vi "launchConnectionListener.vi"(8 "error in (no error)":errorcluster, 11 "BuildServer in":refnum<class "BuildServer.lvclass">) -> (0 "error out":errorcluster, 3 "BuildServer out":refnum<class "BuildServer.lvclass">)   [LabVIEW 2017, in "BuildServer.lvlib" / "BuildServer.lvclass"]
uses:
  BuildServer.lvclass
  C:/Program Files (x86)/National Instruments/LabVIEW 2017/vi.lib/ActorFramework/Actor/Actor.lvclass
  BuildServer.lvclass/BuildServer.ctl
  Communication/Connection Listener/Connection Listener/Connection Listener.lvclass/Connection Listener.ctl
  Communication/Connection Listener/Connection Listener/Read Msg Update.vi
  Communication/Connection Listener/Connection Listener/Connection Listener.lvclass
  <vilib>/ActorFramework/Actor/Actor.lvclass
  Classes/Comm Interface/Comm Interface.lvclass
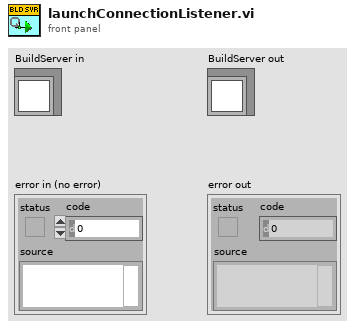
[diagram p1: front panel]
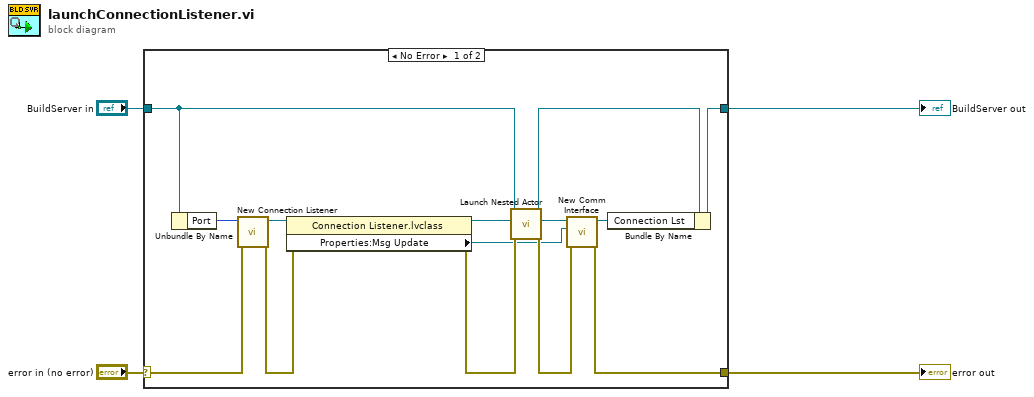
[diagram p0: block diagram]
diagram:
  n1 = case shown="No Error" "error in (no error)" {
    selector: "error in (no error)" -> [w18 w20]
    tunnel: [w10 w20] -> w3
    tunnel: [w14 w19] -> w1
    tunnel: "BuildServer in" -> [w16 w19]
    frame No Error {
      n2 = Unbundle By Name(w16) -> ("Port"=w5:u16)
      n3 = call "New Connection Listener.vi"("error in (no error)"=w18, "Port"=w5) -> ("error out"=w8:errorcluster, "Connection Listener out"=w17:refnum<class "Connection Listener.lvclass">)  [unwired: 8 in]
      n4 = property class="Connection Listener.lvclass"(reference=w17, error in=w8) -> (reference out=w9:refnum<class "Connection Listener.lvclass">, error out=w7:errorcluster, "Properties:Msg Update"=w6:refnum<user-event>)
      n5 = call <vilib>:"Launch Nested Actor.vi"("error in (no error)"=w7, "Nested Actor"=w9, "Caller Actor in"=w16) -> ("error out"=w11:errorcluster, "Nested Actor's Enqueuer"=w13:refnum<class "Message Enqueuer.lvclass">, "Caller Actor out"=w15:refnum<class "BuildServer.lvclass">)  [unwired: 6 in]
      n6 = call "New Comm Interface.vi"("error in (no error)"=w11, "Msg Update"=w6, "Connection Lst Enq"=w13) -> ("error out"=w10:errorcluster, "Comm Interface out"=w12:refnum<class "Comm Interface.lvclass">)  [unwired: 7 in]
      n7 = Bundle By Name(cluster=w15, "Connection Lst"=w12) -> (w14:refnum<class "BuildServer.lvclass">)
    }
    frame Error {
    }
  }
  "error out" <- w3
  "BuildServer out" <- w1
